vi "WS2812 Write Index.vi"() -> ()   [LabVIEW 2017]
uses:
  IMAQCV/PIIO/Core/PIIO DIO.ctl
  IMAQCV/PIIO.lvlib
panel:
  in  "PIN":T1 items=["L1", "L2"]
  in  "Color":u32(colorbox)=16383786
  in  "delay (ms)":u32(slide)=200 scale=0.0..500.0
  in  "stop":bool
  in  "Number of LEDs":u16=40
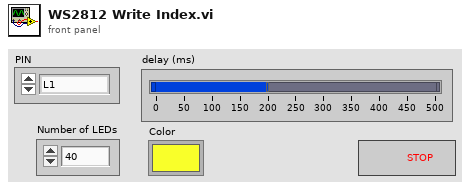
[diagram p1: front panel]
types:
  T1 = typedef "PIIO.lvlib/PIIO DIO.ctl" = u8
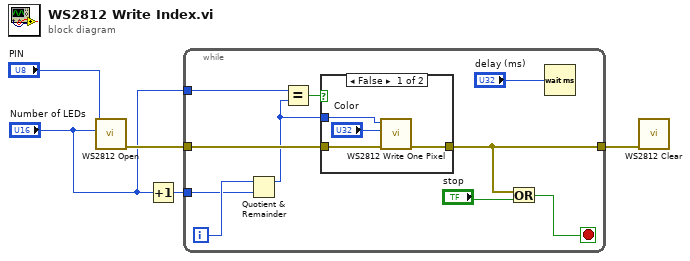
[diagram p0: block diagram]
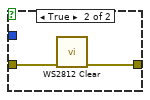
[diagram p2: hidden frame]
diagram:
  n1 = call "WS2812 Open.vi"("Number of LEDs"="Number of LEDs", "PIN"="PIN") -> ("Error Out"=w5:errorcluster)  [unwired: 9 in]
  n2 = Increment(x="Number of LEDs") -> (x+1=w3:u16)
  n3 = while {
    tunnel: w5 -> [w15]
    tunnel: [w12] -> w4
    tunnel: w3 -> [w10]
    tunnel: "Number of LEDs" -> [w7]
    i -> [w14]
    stop <- w11 stop-if-true
    n4 = Quotient & Remainder(x=w14, y=w10) -> (x-y*floor(x/y)=w6:i32)  [unwired: 1 out]
    n5 = Equal?(x=w7, y=w6) -> (x = y?=w8:bool)
    n6 = case shown="False" w8 {
      tunnel: w15 -> [w19 w20]
      tunnel: [w18 w21] -> w12
      tunnel: w6 -> [w16 _]
      frame False {
        n7 = call "WS2812 Write One Pixel.vi"("Error In"=w19, "Color"="Color", "Pixel Index"=w16) -> ("Error Out"=w18:errorcluster)  [unwired: 8 in]
      }
      frame True {
        n8 = call "WS2812 Clear.vi"("Error In"=w20) -> ("Error Out"=w21:errorcluster)  [unwired: 10 in]
      }
    }
    n9 = Or(x=w12, y="stop") -> (x .or. y?=w11:bool)
    n10 = Wait (ms)(milliseconds to wait="delay (ms)") -> ()  [unwired: 1 out]
  }
  n11 = call "WS2812 Clear.vi"("Error In"=w4) -> ()  [unwired: 10 in, 1 out]
